vi "Tool-Kalman Filter - GEN3 raw data.vi"(3 "프런트패널 윈도우:모니터":u16) -> ()   [LabVIEW 2015]
uses:
  SUB_Load and Save Controls.llb/RWC_Actions.ctl
panel:
  in  "Raw data":string
  out "Delta_Filter data":dbl=766.0
  out "Delta_Real GEN3 Data":dbl=766.0
  in  "Export to Excel":bool
  in  "Interval time (ms)":u32=1 min=1 max=5000
  out "Graph":waveform(dbl)[](graph)=[{"t0"=timestamp(3554674983.6106663 s since 1904-01-01), "dt"=11.49265718460083, "Y"=[0.9971512413550824]}, {"t0"=timestamp(3554674983.6106663 s since 1904-01-01), "dt"=11.49265718460083, "Y"=[0.9971599783084714]}]
  in  "Exit":bool
  out "Data Length":i32=766
  in  "R":dbl=0.65 min=0.0 max=1000.0 step=0.1 format="%#.3f"
  in  "Q":dbl=0.004 min=0.0 max=1000.0 step=0.01 format="%#.5f"
  out "Real GEN3 Data":dbl=0.9971512413550824 format="%.5f"
  out "Filter data":dbl=0.9971599783084714 format="%.5f"
  # "CDC Filter Simulation using GEN3 raw data"
  # "Filter Gain setting"
  # "Q: 예측 노이즈 공분산\n    값이 작을수록 무겁게 동작\nR: 측정 노이즈 공분산\n    값이 클수록 무겁게 동작"
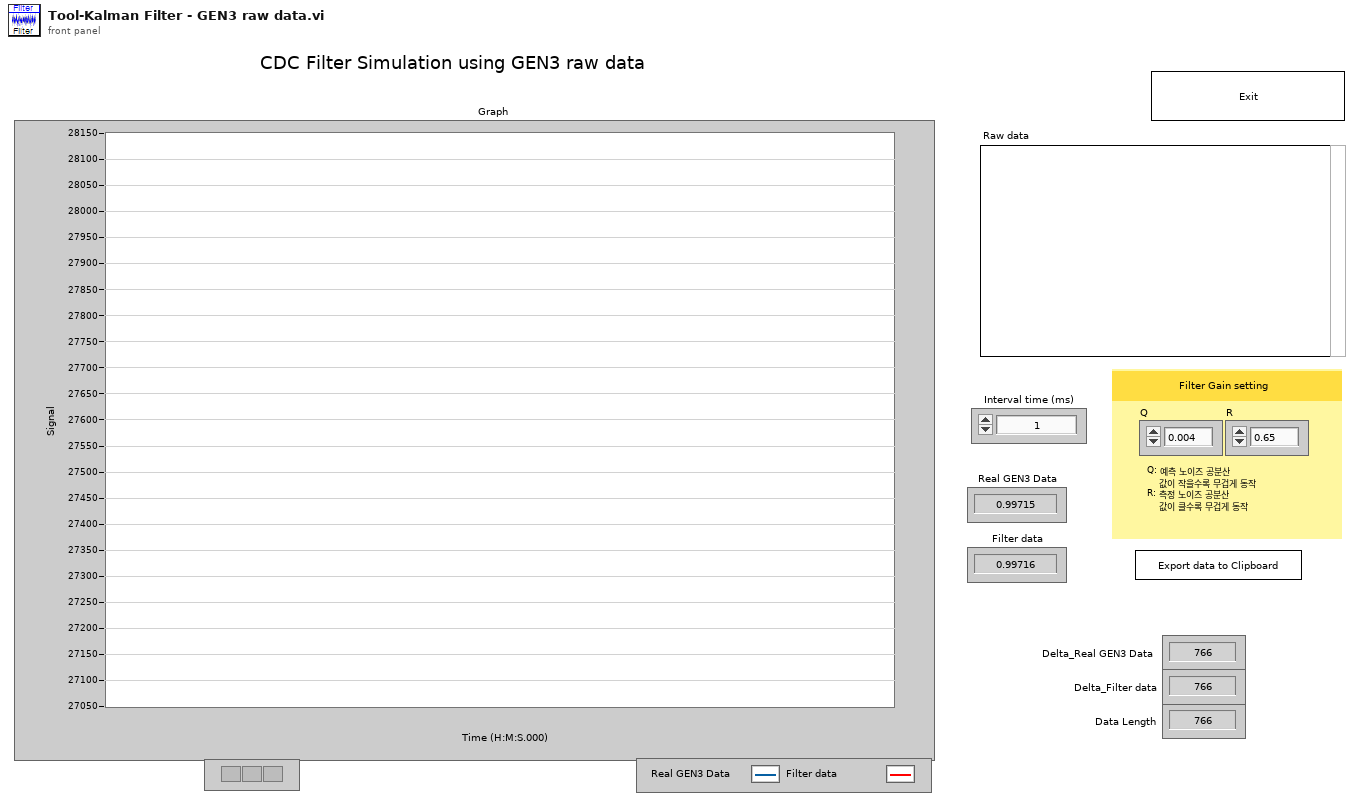
[diagram p1: front panel]
types:
  T1 = typedef "RWC_Actions.ctl" = enum16{"Read", "Write", "Read and Create"}
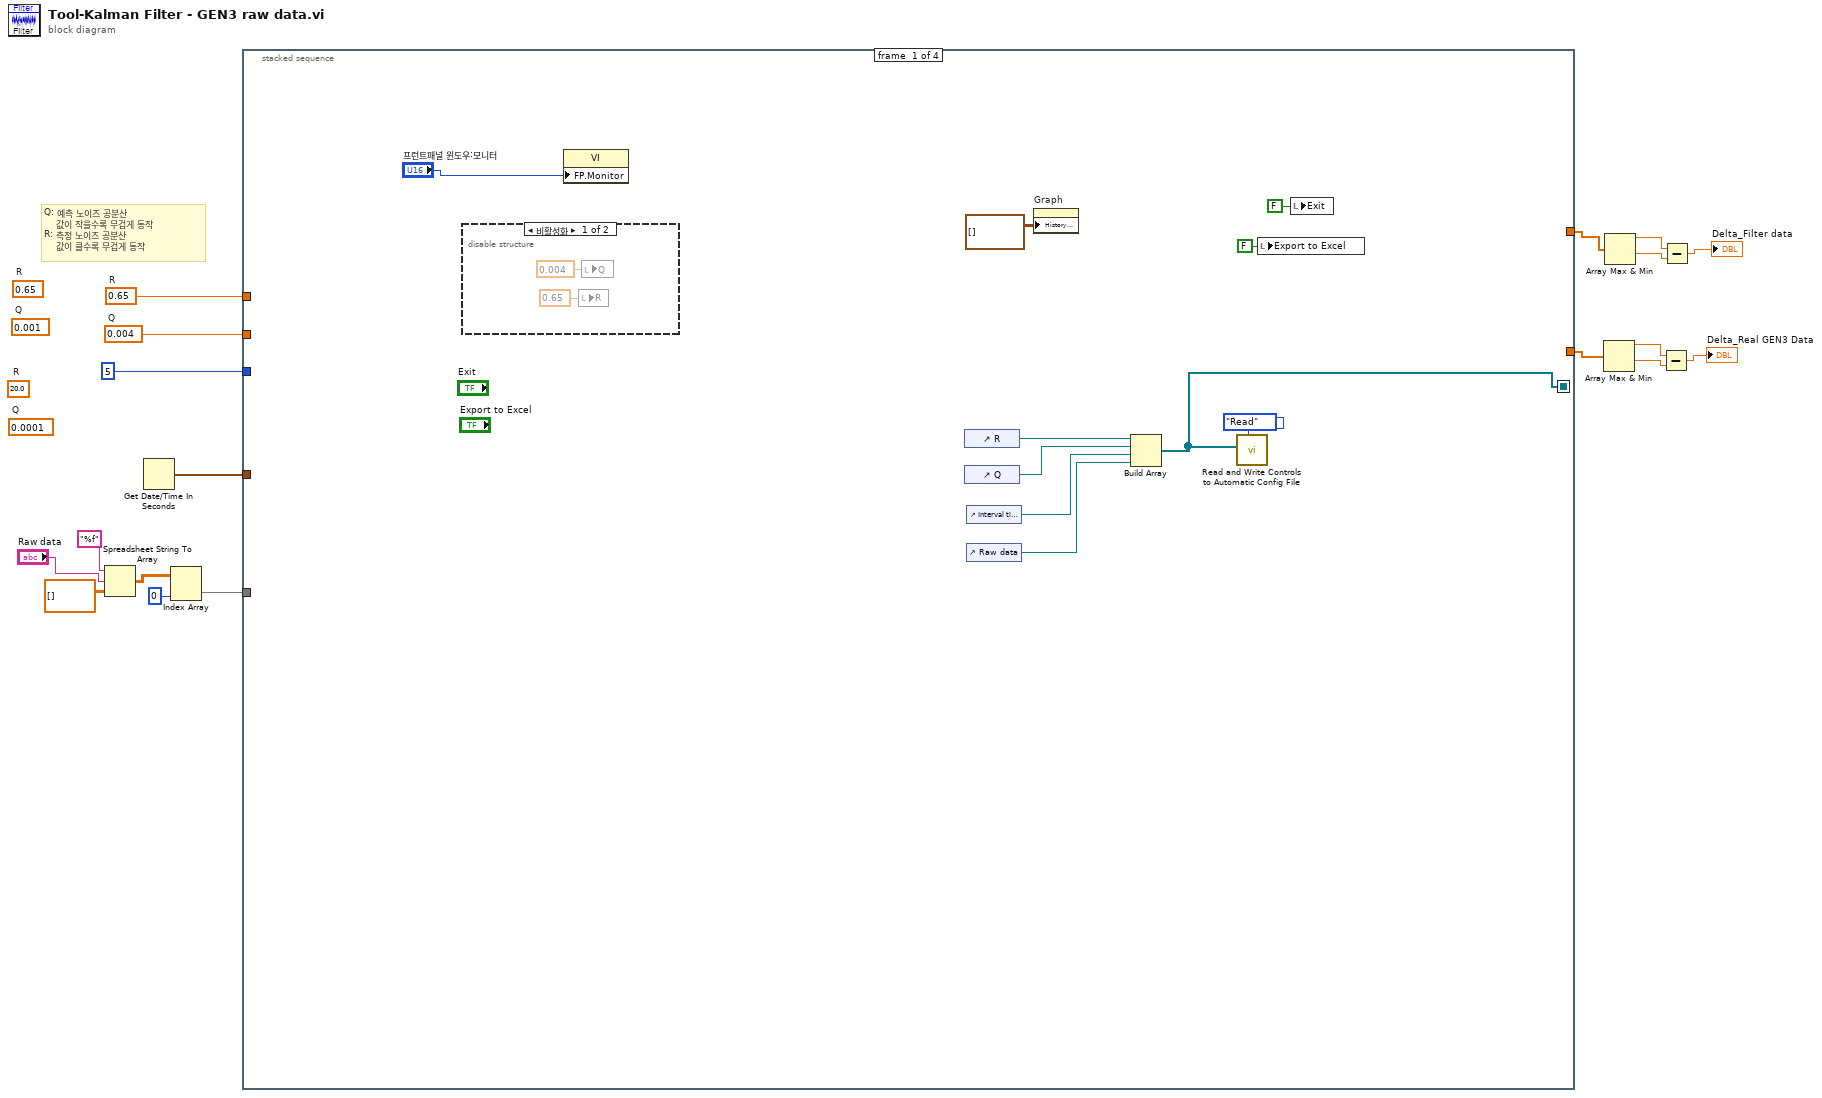
[diagram p0: block diagram]
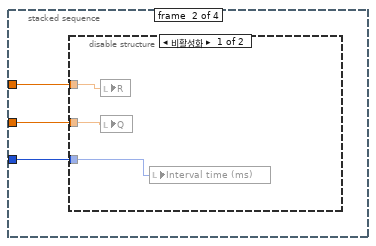
[diagram p3: hidden frame]
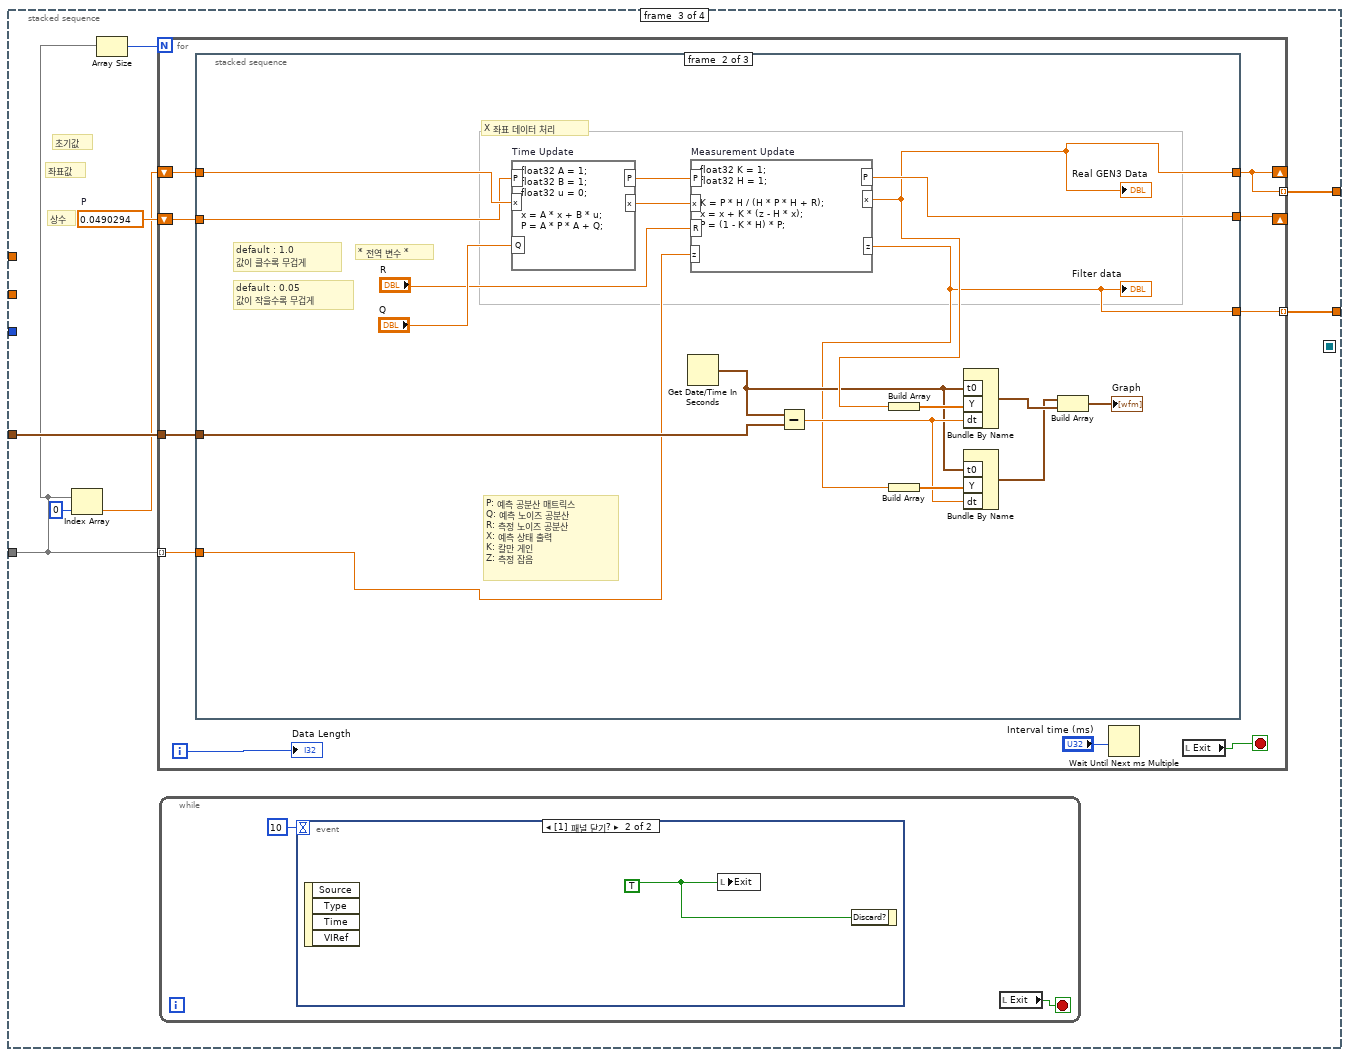
[diagram p5: hidden frame]
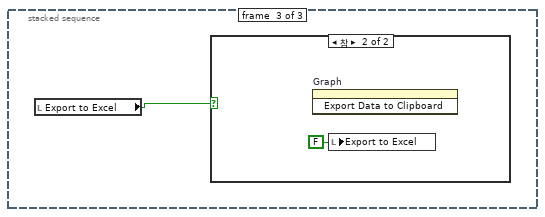
[diagram p7: hidden frame]
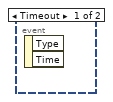
[diagram p9: hidden frame]
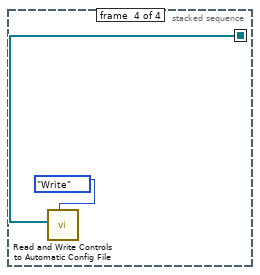
[diagram p10: hidden frame]
diagram:
  (unwired) 0.0001  # Q
  (unwired) 20.0  # R
  (unwired) 0.001  # Q
  (unwired) 0.65  # R
  w11 = 0.004  # Q
  w12 = 0.65  # R
  # "Q: 예측 노이즈 공분산\n    값이 작을수록 무겁게 동작\nR: 측정 노이즈 공분산\n    값이 클수록 무겁게 동작"
  n1 = Spreadsheet String To Array(format string="%f" ("포맷 문자열"), spreadsheet string="Raw data", array type (2D Dbl)=dbl[][] [] ("배열 타입(2D Dbl)")) -> (array=w15:dbl[][])  [unwired: 1 in]
  n2 = Get Date/Time In Seconds() -> (seconds since 1Jan1904=w18:timestamp)
  n3 = Index Array(array=w15, index (col)=0 ("비활성화된 인덱스 (열)")) -> (element=w13:dbl[])  [unwired: 1 in]
  n4 = stacked-sequence {
    seq-local: [w24 _ _ _] -> [_ _ _ w78]
    tunnel: w18 -> [_ _ w43 _]
    tunnel: w13 -> [_ _ w37 _]
    tunnel: w12 -> [_ w33 _ _]
    tunnel: w11 -> [_ w32 _ _]
    tunnel: u32 5 ("Interval time (ms)") -> [_ w31 _ _]
    tunnel: [_ _ w40 _] -> w2
    tunnel: [_ _ w39 _] -> w3
    frame #0 {
      n5 = disable-structure shown="비활성화" {
        frame Disabled {
          n6 = local write "R"(0.65 ("R")) -> ()
          n7 = local write "Q"(0.004 ("Q")) -> ()
        }
        frame Enabled {
        }
      }
      n8 = property class="VI"("FP.Monitor"="프런트패널 윈도우:모니터") -> ()  [unwired: 2 in, 2 out]
      n9 = control-ref of="R"() -> (w23:refnum<vi>)
      n10 = control-ref of="Q"() -> (w22:refnum<vi>)
      n11 = control-ref of="Interval time (ms)"() -> (w21:refnum<vi>)
      n12 = control-ref of="Raw data"() -> (w19:refnum<vi>)
      n13 = property on="Graph" class="WFChart (엄격한)"("History Data"=waveform(dbl)[][] [] ("히스토리 데이터")) -> ()  [unwired: 2 in, 2 out]
      n14 = Build Array(w23, w22, w21, w19) -> (w24:refnum<vi>[])
      n15 = call "Read and Write Controls to Automatic Config File.vi"("Action"=RWC_Actions."Read", "Control References"=w24) -> ()  [unwired: 9 in, 1 out]
      n16 = local write "Export to Excel"(FALSE ("Export to Excel")) -> ()
      n17 = local write "Exit"(FALSE ("Exit")) -> ()
    }
    frame #1 {
      n18 = disable-structure shown="비활성화" {
        disable-tunnel: w33 -> [w36 _]
        disable-tunnel: w32 -> [w35 _]
        disable-tunnel: w31 -> [w34 _]
        frame Disabled {
          n19 = local write "R"(w36) -> ()
          n20 = local write "Q"(w35) -> ()
          n21 = local write "Interval time (ms)"(w34) -> ()
        }
        frame Enabled {
        }
      }
    }
    frame #2 {
      w44 = 0.0490294  # P
      # "좌표값"
      # "상수"
      # "초기값"
      n22 = Index Array(array=w37, index=0 ("인덱스")) -> (element=w41:dbl)
      n23 = Array Size(array=w37) -> (size(s)=w38:i32)
      n24 = for {
        N: w38 -> [_]
        shift-right: [w47] -> _
        shift-left: w41 -> [w53]
        shift-right: [w52] -> _
        shift-left: w44 -> [w54]
        tunnel: w43 -> [w51]
        tunnel: w37 -> [w48] mode=indexing
        tunnel: [w47] -> w40 mode=indexing
        tunnel: [w46] -> w39 mode=indexing
        i -> [w50]
        stop <- w45 stop-if-true
        n25 = stacked-sequence {
          tunnel: w54 -> [_ w67 _]
          tunnel: w53 -> [_ w72 _]
          tunnel: [_ w71 _] -> w52
          tunnel: [_ w70 _] -> w47
          tunnel: w51 -> [_ w66 _]
          tunnel: w48 -> [_ w65 _]
          tunnel: [_ w55 _] -> w46
          frame #0 {
          }
          frame #1 {
            # "P: 예측 공분산 매트릭스\nQ: 예측 노이즈 공분산\nR: 측정 노이즈 공분산\nX: 예측 상태 출력 \nK: 칼만 게인\nZ: 측정 잡음"
            # "X 좌표 데이터 처리"
            # "* 전역 변수 *"
            # "default : 0.05\n값이 작을수록 무겁게"
            # "default : 1.0\n값이 클수록 무겁게"
            n26 = formula code="float32 A = 1;\nfloat32 B = 1;\nfloat32 u = 0;\n\nx = A * x + B * u;\nP = A * P * A + Q;" "Time Update"("x"=w72, "P"=w67, "Q"="Q") -> ("x"=w64:dbl, "P"=w63:dbl)
            n27 = Get Date/Time In Seconds() -> (seconds since 1Jan1904=w56:timestamp)
            n28 = formula code="float32 K = 1;\nfloat32 H = 1;\n\nK = P * H / (H * P * H + R);\nx = x + K * (z - H * x);\nP = (1 - K * H) * P;" "Measurement Update"("x"=w64, "P"=w63, "z"=w65, "R"="R") -> ("x"=w70:dbl, "P"=w71:dbl, "z"=w55:dbl)
            "Real GEN3 Data" <- w70
            "Filter data" <- w55
            n29 = Subtract(x=w56, y=w66) -> (x-y=w59:dbl)
            n30 = Build Array(w70) -> (w62:dbl[])
            n31 = Build Array(w55) -> (w61:dbl[])
            n32 = Bundle By Name("t0"=w56, "Y"=w62, "dt"=w59) -> (w60:waveform(dbl))  [unwired: 1 in]
            n33 = Bundle By Name("t0"=w56, "Y"=w61, "dt"=w59) -> (w58:waveform(dbl))  [unwired: 1 in]
            n34 = Build Array(w58, w60) -> (→"Graph":waveform(dbl)[])
          }
          frame #2 {
            n35 = local read "Export to Excel"() -> (w73:bool)
            n36 = case shown="참" w73 {
              frame False {
              }
              frame True {
                n37 = invoke on="Graph" class="WFChart (엄격한)" method="Export Data to Clipboard"() -> ()  [unwired: 3 in, 3 out]
                n38 = local write "Export to Excel"(FALSE ("Export to Excel")) -> ()
              }
            }
          }
        }
        n39 = Wait Until Next ms Multiple(millisecond multiple="Interval time (ms)") -> ()  [unwired: 1 out]
        n40 = local read "Exit"() -> (w45:bool)
        "Data Length" <- w50
      }
      n41 = while {
        stop <- w75 stop-if-true
        n42 = event shown="[1] 패널 닫기?" {
          selector: _ -> [_ _]
          dyn-events: _ -> [_ _]
          timeout: 10 -> [_ _]
          event Timeout {
            n43 = event-data() -> ()  [unwired: 1 in, 2 out]
          }
          event Panel Close? {
            w77 = TRUE ("Exit")
            n44 = event-data() -> ()  [unwired: 1 in, 4 out]
            n45 = local write "Exit"(w77) -> ()
            n46 = event-data("Discard?"=w77) -> ()  [unwired: 1 in, 1 out]
          }
        }
        n47 = local read "Exit"() -> (w75:bool)
      }
    }
    frame #3 {
      n48 = call "Read and Write Controls to Automatic Config File.vi"("Action"=RWC_Actions."Write", "Control References"=w78) -> ()  [unwired: 9 in, 1 out]
    }
  }
  n49 = Array Max & Min(array=w3) -> (max value=w9:dbl, min value=w8:dbl)  [unwired: 2 out]
  n50 = Array Max & Min(array=w2) -> (max value=w5:dbl, min value=w6:dbl)  [unwired: 2 out]
  n51 = Subtract(x=w9, y=w8) -> (x-y=→"Delta_Real GEN3 Data":dbl)
  n52 = Subtract(x=w5, y=w6) -> (x-y=→"Delta_Filter data":dbl)
